vi "StartStop.vi"(8 "error in (no error)":errorcluster, 10 "Start/Stop":bool, 11 "Generador de Señales in":refnum<class "Generador de Señales.lvclass">) -> (0 "error out":errorcluster, 3 "Generador de Señales out":refnum<class "Generador de Señales.lvclass">)   [LabVIEW 2020, in "Generador de Señales.lvlib" / "Generador de Señales.lvclass"]
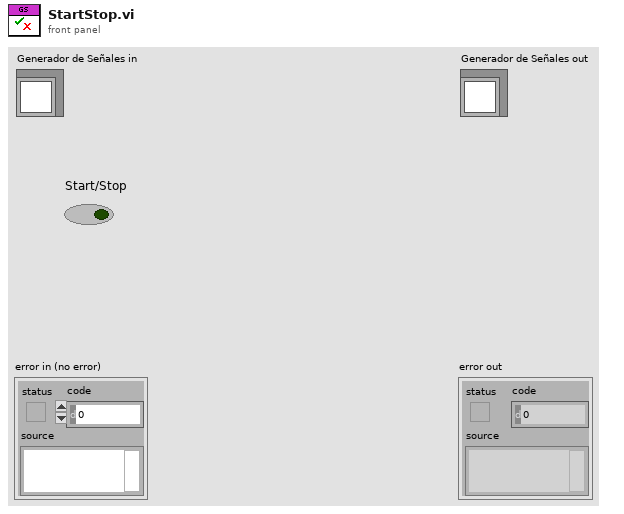
[diagram p1: front panel]
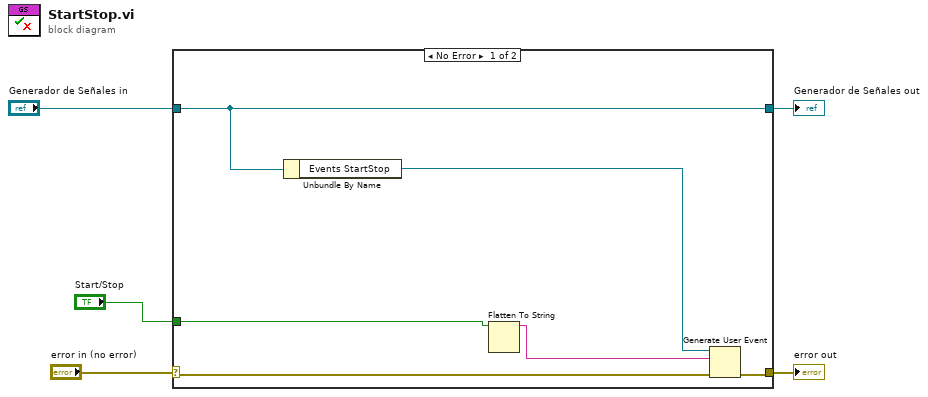
[diagram p0: block diagram]
diagram:
  n1 = case shown="No Error" "error in (no error)" {
    selector: "error in (no error)" -> [w10 w13]
    tunnel: [w11 w13] -> w4
    tunnel: [w9 w12] -> w2
    tunnel: "Generador de Señales in" -> [w9 w12]
    tunnel: "Start/Stop" -> [w7 _]
    frame No Error {
      n2 = Unbundle By Name(w9) -> ("Events StartStop"=w8:refnum<user-event>)
      n3 = Flatten To String(anything=w7) -> (data string=w6:string)  [unwired: 3 in, 2 out]
      n4 = Generate User Event(user event=w8, event data cluster=w6, error in=w10) -> (error out=w11:errorcluster)  [unwired: 1 in, 1 out]
    }
    frame Error {
    }
  }
  "error out" <- w4
  "Generador de Señales out" <- w2
